vi "Write Key (Variant)__ogtk.vi"(5 "float number format":string, 6 "write raw string? (F)":bool, 7 "section":string, 8 "error in (no error)":errorcluster, 9 "key-value":variant, 10 "key (optional)":string, 11 "refnum":T1) -> (0 "error out":errorcluster, 3 "refnum out":T1)   [LabVIEW 2020]
doc: "Writes a value associated with key in a specified section of the configuration data identified by refnum. If \"key\" input is not specified, the name of the variant object is used as the key.\n\nFor example a Boolean named \"Enable\" with a value of TRUE would correspond to the key-value pair:\n\nEnable=TRUE\n\nNote: Special characters in section and key names will be escape-coded. These include the following: \\00-\\1F (non-printable chars); \"[\", \"]\", and \"=\" (INI syntax elements); \\FE (\"þ\") and \\FF (\"ÿ\") (legacy bracket encoding); Additionally, the escape character, \"\\\", will be escaped as \"\\\\\"."
uses:
  <vilib>/Utility/config.llb/Config Data RefNum.ctl
  <vilib>/Utility/config.llb/Write Key (String).vi
  <vilib>/Utility/config.llb/Write Key (Path).vi
  <vilib>/Utility/config.llb/NI_LVConfig.lvlib
panel:
  in  "Ref for recursive call":refnum<vi>
  # "Write Key (Variant).vi\n\nWrites a variant key-value to INI file.\n\nPlease visit http://www.OpenG.org to learn about the\nOpen Source LabVIEW software movement.\n\nNOTICE -- YOU MUST LEAVE THIS NOTICE IN PLACE.  PER THE TERMS OF THE LICENSE BELOW, YOU MAY SUBLICENSE THIS SOFTWARE \nIN ANY WAY THAT DOES NOT CONFLICT WITH THIS LICENSE.\n\n### BSD License (http://www.opensource.org/licenses/bsd-license.php) Begin ###\n \nCopyright (c) 2002, Jean-Pierre Drolet <drolet_jp@hotmail.com>\nCopyright (c) 2002-2006, Jim Kring <jim@jimkring.com>\n\nAll rights reserved.\n\nRedistribution and use in source and binary forms, with or without modification, are permitted provided that the following conditions are met:\n\n    * Redistributions of source code must retain the above copyright notice, this list of conditions and the following disclaimer.\n    * Redistributions in binary form must reproduce the above copyright notice, this list of conditions and the following disclaimer in the \n       documentation and/or other materials provided with the distribution.\n    * Neither the name of SciWare, James Kring, Inc., nor the names of its contributors may be used to endorse or promote products derived \n       from this software without specific prior written permission.\n\nTHIS SOFTWARE IS PROVIDED BY THE COPYRIGHT HOLDERS AND CONTRIBUTORS \"AS IS\" AND ANY EXPRESS OR IMPLIED WARRANTIES, \nINCLUDING, BUT NOT LIMITED TO, THE IMPLIED WARRANTIES OF MERCHANTABILITY AND FITNESS FOR A PARTICULAR PURPOSE ARE \nDISCLAIMED. IN NO EVENT SHALL THE COPYRIGHT OWNER OR CONTRIBUTORS BE LIABLE FOR ANY DIRECT, INDIRECT, INCIDENTAL,\n SPECIAL, EXEMPLARY, OR CONSEQUENTIAL DAMAGES (INCLUDING, BUT NOT LIMITED TO, PROCUREMENT OF SUBSTITUTE GOODS OR \nSERVICES; LOSS OF USE, DATA, OR PROFITS; OR BUSINESS INTERRUPTION) HOWEVER CAUSED AND ON ANY THEORY OF LIABILITY, \nWHETHER IN CONTRACT, STRICT LIABILITY, OR TORT (INCLUDING NEGLIGENCE OR OTHERWISE) ARISING IN ANY WAY OUT OF THE USE \nOF THIS SOFTWARE, EVEN IF ADVISED OF THE POSSIBILITY OF SUCH DAMAGE.\n\n### BSD License End ###"
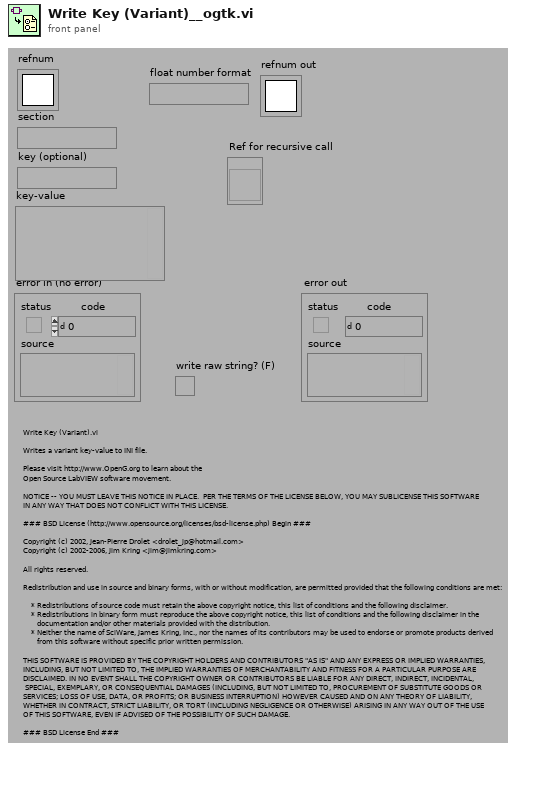
[diagram p1: front panel]
types:
  T1 = typedef "NI_LVConfig.lvlib/Config Data RefNum.ctl" = refnum<k1>
  T2 = typedef "Type Descriptor Enumeration__ogtk.ctl" = enum8{"<Null>", "I8", "I16", "I32", "I64", "U8", "U16", "U32", "U64", "SGL", "DBL", "EXT", "CSG", "CDB", "CXT", "0x0F", "0x10", "0x11", "0x12", "0x13", "0x14", "Enum U8", "Enum U16", "Enum U32", "Enum U64", "SGL PQ", "DBL PQ", "EXT PQ", "CSG PQ", "CDB PQ", "CXT PQ", "0x1F", "0x20", "Boolean", "0x22", "0x23", "0x24", "0x25", "0x26", "0x27", "0x28", "0x29", "0x2A", "0x2B", "0x2C", "0x2D", "0x2E", "0x2F", "String", "0x31", "Path", "Pict", "0x34", "0x35", "0x36", "DAQ", "0x38", "0x39", "0x3A", "0x3B", "0x3C", "0x3D", "0x3E", "0x3F", "Array", "0x41", "0x42", "0x43", "0x44", "0x45", "0x46", "0x47", "0x48", "0x49", "0x4A", "0x4B", "0x4C", "0x4D", "0x4E", "0x4F", "Cluster", "0x51", "0x52", "Variant", "Waveform", "0x55", "0x56", "0x57", "0x58", "0x59", "0x5A", "0x5B", "0x5C", "0x5D", "0x5E", "Fixed Point", "0x60", "0x61", "0x62", "0x63", "0x64", "0x65", "0x66", "0x67", "0x68", "0x69", "0x6A", "0x6B", "0x6C", "0x6D", "0x6E", "0x6F", "Refnum", "0x71", "0x72", "Set Collection", "Map Collection"}
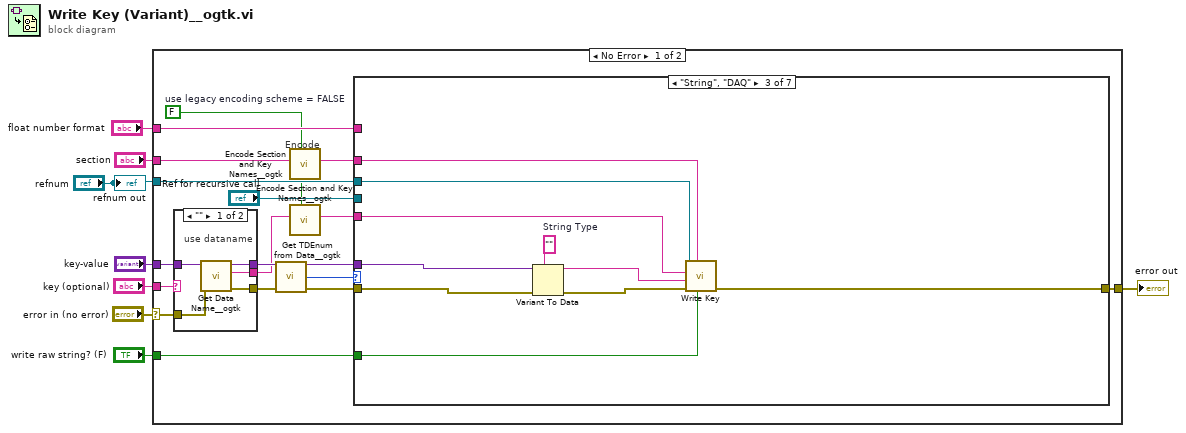
[diagram p0: block diagram]
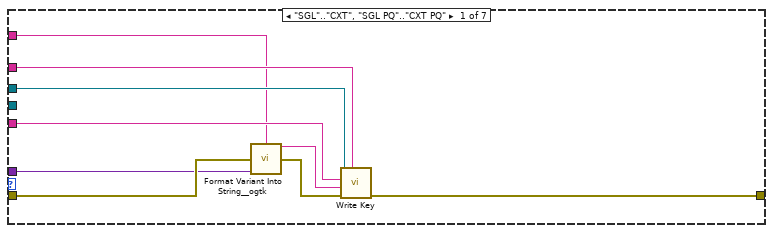
[diagram p2: hidden frame]
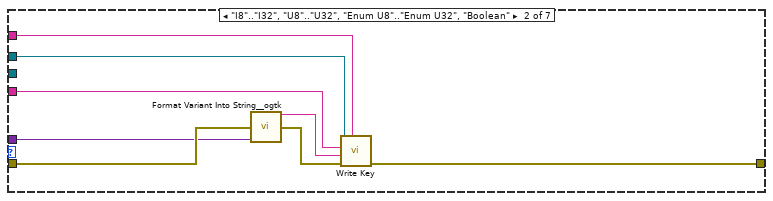
[diagram p3: hidden frame]
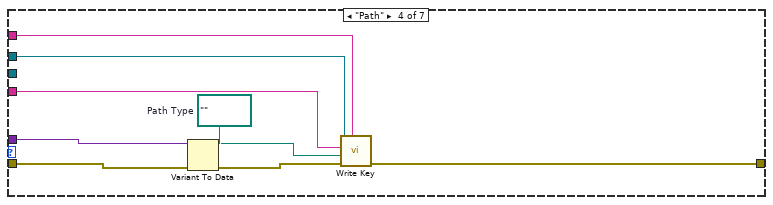
[diagram p4: hidden frame]
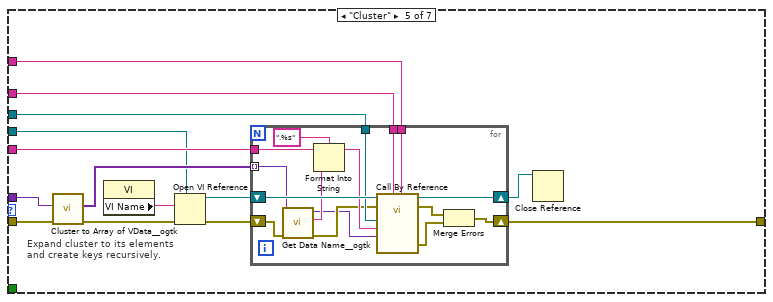
[diagram p5: hidden frame]
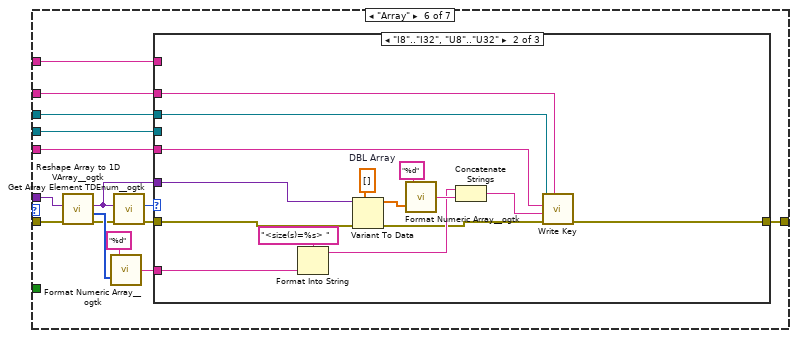
[diagram p6: hidden frame]
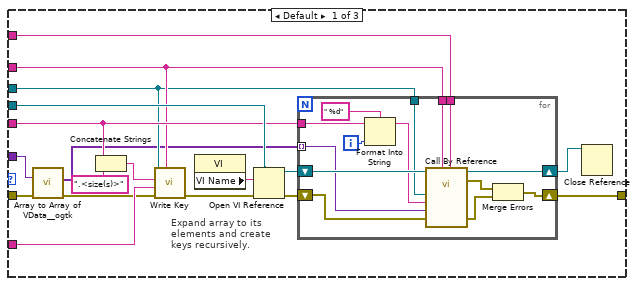
[diagram p7: hidden frame]
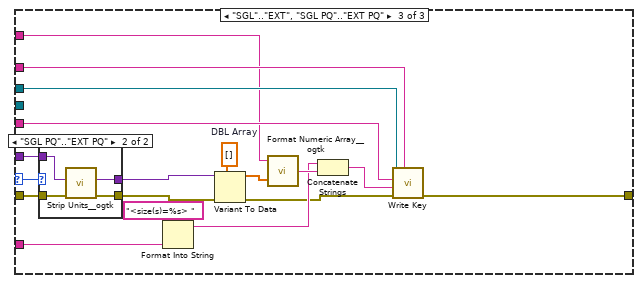
[diagram p8: hidden frame]
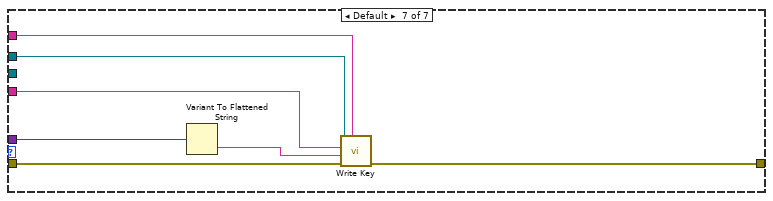
[diagram p10: hidden frame]
diagram:
  n1 = case shown="No Error" "error in (no error)" {
    selector: "error in (no error)" -> [w21 w192]
    tunnel: "refnum" -> [w24 _]
    tunnel: [w23 w192] -> w8
    tunnel: "key-value" -> [w18 _]
    tunnel: "key (optional)" -> [w22 _]
    tunnel: "section" -> [w13 _]
    tunnel: "float number format" -> [w15 _]
    tunnel: "write raw string? (F)" -> [w14 _]
    frame No Error {
      w9 = FALSE  # use legacy encoding scheme = FALSE
      # "Encode"
      n2 = case shown="\"\"" w22 {
        selector: w22 -> [_ w191]
        tunnel: [w188 w191] -> w11
        tunnel: w18 -> [w185 w189]
        tunnel: w21 -> [w187 w190]
        tunnel: [w186 w190] -> w19
        tunnel: [w184 w189] -> w17
        frame "" {
          # "use dataname"
          n3 = call <userlib>:"Get Data Name__ogtk.vi"("error in (no error)"=w187, "Data"=w185) -> ("error out"=w186:errorcluster, "Data Name"=w188:string, "Data dup"=w184:variant)  [unwired: 7 in]
        }
        frame Default {
          # "use optional\nkey"
        }
      }
      n4 = call <userlib>:"Get TDEnum from Data__ogtk.vi"("Data"=w17) -> ("Type Descriptor Enumeration"=w20:T2)  [unwired: 4 in]
      n5 = call <userlib>:"Encode Section and Key Names__ogtk.vi"("use legacy encoding scheme? (FALSE)"=w9, "string"=w13) -> ("encoded string"=w12:string)  [unwired: 9 in]
      n6 = call <userlib>:"Encode Section and Key Names__ogtk.vi"("use legacy encoding scheme? (FALSE)"=w9, "string"=w11) -> ("encoded string"=w10:string)  [unwired: 9 in]
      n7 = case shown="\"String\", \"DAQ\"" w20 {
        tunnel: w17 -> [w28 w36 w49 w58 w67 w103 w179]
        tunnel: w24 -> [w33 w41 w48 w57 w71 w97 w183]
        tunnel: [w32 w40 w46 w55 w69 w105 w182] -> w23
        tunnel: w19 -> [w29 w37 w45 w54 w66 w102 w178]
        tunnel: w10 -> [w31 w39 w44 w53 w63 w96 w181]
        tunnel: w12 -> [w30 w38 w43 w52 w70 w98 w180]
        tunnel: "Ref for recursive call" -> [_ _ _ _ w62 w104 _]
        tunnel: w15 -> [w27 _ _ _ w61 w91 _]
        tunnel: w14 -> [_ _ w42 _ _ _ _]
        frame "SGL".."CXT", "SGL PQ".."CXT PQ" {
          n8 = call <userlib>:"Format Variant Into String__ogtk.vi"("Format String"=w27, "error in (no error)"=w29, "Variant"=w28) -> ("Output String"=w25:string, "error out"=w26:errorcluster)  [unwired: 11 in]
          n9 = call-poly <vilib>:"Write Key.vi"("section"=w30, "error in (no error)"=w26, "value"=w25, "key"=w31, "refnum"=w33) -> ("error out"=w32:errorcluster)  [unwired: 4 in, 2 out]
        }
        frame "I8".."I32", "U8".."U32", "Enum U8".."Enum U32", "Boolean" {
          n10 = call <userlib>:"Format Variant Into String__ogtk.vi"("error in (no error)"=w37, "Variant"=w36) -> ("Output String"=w34:string, "error out"=w35:errorcluster)  [unwired: 12 in]
          n11 = call-poly <vilib>:"Write Key.vi"("section"=w38, "error in (no error)"=w35, "value"=w34, "key"=w39, "refnum"=w41) -> ("error out"=w40:errorcluster)  [unwired: 4 in, 2 out]
        }
        frame "String", "DAQ" {
          w51 = ""  # String Type
          n12 = Variant To Data(error in=w45, type=w51, Variant=w49) -> (data=w50:string, error out=w47:errorcluster)
          n13 = call-poly <vilib>:"Write Key.vi"("write raw string? (F)"=w42, "section"=w43, "error in (no error)"=w47, "value"=w50, "key"=w44, "refnum"=w48) -> ("error out"=w46:errorcluster)  [unwired: 3 in, 2 out]
        }
        frame "Path" {
          w60 = path ""  # Path Type
          n14 = Variant To Data(error in=w54, type=w60, Variant=w58) -> (data=w59:path, error out=w56:errorcluster)
          n15 = call-poly <vilib>:"Write Key.vi"("section"=w52, "error in (no error)"=w56, "value"=w59, "key"=w53, "refnum"=w57) -> ("error out"=w55:errorcluster)  [unwired: 4 in, 2 out]
        }
        frame "Cluster" {
          # "Expand cluster to its elements\nand create keys recursively."
          n16 = call <userlib>:"Cluster to Array of VData__ogtk.vi"("error in (no error)"=w66, "Cluster"=w67) -> ("error out"=w64:errorcluster, "Array of VData"=w65:variant[])  [unwired: 8 in]
          n17 = property class="VI"() -> ("VI Name"=w68:string)  [unwired: 2 in, 2 out]
          n18 = Open VI Reference(type specifier VI Refnum (for type only)=w62, vi path=w68, error in (no error)=w64) -> (vi reference=w74:refnum<vi>, error out=w72:errorcluster)  [unwired: 3 in]
          n19 = for {
            shift-right: [w89] -> w73
            shift-left: w74 -> [w90]
            shift-right: [w84] -> w69
            shift-left: w72 -> [w79]
            tunnel: w65 -> [w77] mode=indexing
            tunnel: w70 -> [w88]
            tunnel: w71 -> [w87]
            tunnel: w63 -> [w83]
            tunnel: w61 -> [w75]
            n20 = call <userlib>:"Get Data Name__ogtk.vi"("error in (no error)"=w79, "Data"=w77) -> ("error out"=w78:errorcluster, "Data Name"=w82:string, "Data dup"=w76:variant)  [unwired: 7 in]
            n21 = Format Into String(format string=".%s" ("Format String"), initial string=w83, w82) -> (resulting string=w81:string)  [unwired: 1 in, 1 out]
            n22 = call-by-ref "?"(reference=w90, error in=w78, "format string"=w75, "section"=w88, "key-value"=w76, "key (optional)"=w81, "refnum"=w87) -> (reference out=w89:refnum<vi>, error out=w85:errorcluster, "error out"=w86:errorcluster)  [unwired: 5 in, 1 out]
            n23 = Merge Errors(w85, w86) -> (w84:errorcluster)
          }
          n24 = Close Reference(reference=w73) -> ()  [unwired: 1 in, 1 out]
        }
        frame "Array" {
          n25 = call <userlib>:"Reshape Array to 1D VArray__ogtk.vi"("error in (no error)"=w102, "MultiD Array"=w103) -> ("error out"=w92:errorcluster, "Size(s)"=w100:u32[], "1D VArray"=w93:variant)  [unwired: 7 in]
          n26 = call <userlib>:"Format Numeric Array__ogtk.vi"("Array"=w100, "format string"="%d") -> ("Formatted on a line"=w94:string)
          n27 = call <userlib>:"Get Array Element TDEnum__ogtk.vi"("error in (no error)"=w92, "Array"=w93) -> ("error out"=w95:errorcluster, "Element Type"=w99:T2)  [unwired: 8 in]
          n28 = case shown="\"I8\"..\"I32\", \"U8\"..\"U32\"" w99 {
            selector: w99 -> [_ _ w158]
            tunnel: w97 -> [w113 w141 w161]
            tunnel: w98 -> [w114 w142 w162]
            tunnel: [w120 w139 w159] -> w105
            tunnel: w96 -> [w117 w140 w160]
            tunnel: w104 -> [w118 _ _]
            tunnel: w95 -> [w110 w143 w157]
            tunnel: w94 -> [w111 w144 w163]
            tunnel: w93 -> [w108 w138 w155]
            tunnel: w91 -> [w106 _ w153]
            frame Default {
              # "Expand array to its\nelements and create\nkeys recursively."
              n29 = call <userlib>:"Array to Array of VData__ogtk.vi"("error in (no error)"=w110, "MultiD Array"=w108) -> ("error out"=w109:errorcluster, "1D Array of Variants"=w107:variant[])  [unwired: 8 in]
              n30 = Concatenate Strings(w117, ".<size(s)>" ("Substring")) -> (w112:string)
              n31 = call-poly <vilib>:"Write Key.vi"("section"=w114, "error in (no error)"=w109, "value"=w111, "key"=w112, "refnum"=w113) -> ("error out"=w116:errorcluster)  [unwired: 4 in, 2 out]
              n32 = property class="VI"() -> ("VI Name"=w119:string)  [unwired: 2 in, 2 out]
              n33 = Open VI Reference(type specifier VI Refnum (for type only)=w118, vi path=w119, error in (no error)=w116) -> (vi reference=w123:refnum<vi>, error out=w121:errorcluster)  [unwired: 3 in]
              n34 = for {
                shift-right: [w136] -> w122
                shift-left: w123 -> [w137]
                shift-right: [w131] -> w120
                shift-left: w121 -> [w126]
                tunnel: w107 -> [w127] mode=indexing
                tunnel: w114 -> [w135]
                tunnel: w113 -> [w134]
                tunnel: w117 -> [w130]
                tunnel: w106 -> [w124]
                i -> [w125]
                n35 = Format Into String(format string=" %d" ("Format String"), initial string=w130, w125) -> (resulting string=w129:string)  [unwired: 1 in, 1 out]
                n36 = call-by-ref "?"(reference=w137, "format string"=w124, "section"=w135, "error in (no error)"=w126, "key-value"=w127, "key (optional)"=w129, "refnum"=w134) -> (reference out=w136:refnum<vi>, error out=w132:errorcluster, "error out"=w133:errorcluster)  [unwired: 5 in, 1 out]
                n37 = Merge Errors(w132, w133) -> (w131:errorcluster)
              }
              n38 = Close Reference(reference=w122) -> ()  [unwired: 1 in, 1 out]
            }
            frame "I8".."I32", "U8".."U32" {
              w152 = dbl[] []  # DBL Array
              n39 = Format Into String(format string="<size(s)=%s> " ("Format String"), w144) -> (resulting string=w147:string)  [unwired: 2 in, 1 out]
              n40 = Variant To Data(error in=w143, type=w152, Variant=w138) -> (data=w151:dbl[], error out=w146:errorcluster)
              n41 = call <userlib>:"Format Numeric Array__ogtk.vi"("Array"=w151, "format string"="%d") -> ("Formatted on a line"=w150:string)
              n42 = Concatenate Strings(w147, w150) -> (w145:string)
              n43 = call-poly <vilib>:"Write Key.vi"("section"=w142, "error in (no error)"=w146, "value"=w145, "key"=w140, "refnum"=w141) -> ("error out"=w139:errorcluster)  [unwired: 4 in, 2 out]
            }
            frame "SGL".."EXT", "SGL PQ".."EXT PQ" {
              w170 = dbl[] []  # DBL Array
              n44 = case shown="\"SGL PQ\"..\"EXT PQ\"" w158 {
                tunnel: w157 -> [w172 w176]
                tunnel: [w172 w175] -> w156
                tunnel: w155 -> [w171 w174]
                tunnel: [w171 w173] -> w154
                frame Default {
                }
                frame "SGL PQ".."EXT PQ" {
                  n45 = call <userlib>:"Strip Units__ogtk.vi"("error in (no error)"=w176, "Number or 1D array with units"=w174) -> ("error out"=w175:errorcluster, "Pure Number(s) (base units)"=w173:variant)  [unwired: 8 in]
                }
              }
              n46 = Format Into String(format string="<size(s)=%s> " ("Format String"), w163) -> (resulting string=w166:string)  [unwired: 2 in, 1 out]
              n47 = Variant To Data(error in=w156, type=w170, Variant=w154) -> (data=w169:dbl[], error out=w165:errorcluster)
              n48 = call <userlib>:"Format Numeric Array__ogtk.vi"("Array"=w169, "format string"=w153) -> ("Formatted on a line"=w168:string)
              n49 = Concatenate Strings(w166, w168) -> (w164:string)
              n50 = call-poly <vilib>:"Write Key.vi"("section"=w162, "error in (no error)"=w165, "value"=w164, "key"=w160, "refnum"=w161) -> ("error out"=w159:errorcluster)  [unwired: 4 in, 2 out]
            }
          }
        }
        frame Default {
          n51 = Variant To Flattened String(Variant=w179) -> (data string=w177:string)  [unwired: 1 out]
          n52 = call-poly <vilib>:"Write Key.vi"("section"=w180, "error in (no error)"=w178, "value"=w177, "key"=w181, "refnum"=w183) -> ("error out"=w182:errorcluster)  [unwired: 4 in, 2 out]
        }
      }
    }
    frame Error {
    }
  }
  "error out" <- w8
  "refnum out" <- "refnum"
